vi "Version 1_Write Tare Settings.vi"(6 "Totalizer Timer":enum32{"Disable", "Enable", "No Change"}(radio)=enum."No Change", 8 "error in":errorcluster, 9 "ValveDrive Report":enum32{"Disable", "Enable", "No Change"}(radio)=enum."No Change", 10 "Tare Functions":T1={"Display"=enum."None", "External"=enum."None", "Auto Delay"=nan} {"Auto Delay" format="%.1g"}, 11 "VISA Session In":refnum<visa-resource-name>="Alicat") -> (0 "error out":errorcluster, 3 "VISA Session Out":refnum<visa-resource-name>)   [LabVIEW 2015]
panel:
  in  "Address (A)":string="A"
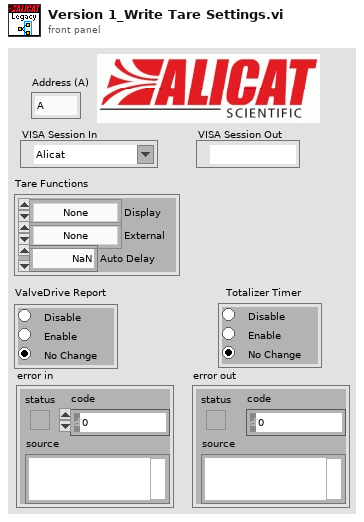
[diagram p1: front panel]
types:
  T1 = cluster{"Display":enum16{"None", "Pressure", "Volumetric"}, "External":enum16{"None", "Pressure", "Volumetric", "Totalizer"}, "Auto Delay":dbl}
  T2 = cluster{"Valve Drive":bool, "Totalizer":bool, "Totalizer Timer":bool, "Totalizer Peak Flow":bool, "Show Abs., Gauge\nand Baro. pressures":bool}
  T3 = cluster{"Pressure(s)":bool, "Temperature":bool, "Volumetric":bool, "Mass":bool, "Totalizer Average Flow":bool, "Gas Selected":bool}
  T4 = cluster{"Absolute Pressure":bool, "Gauge/Diff. Pressure":bool, "Barometric Pressure":bool, "Temperature":bool, "Volumetric":bool, "Mass":bool, "Setpoint":bool, "Valve Drive":bool, "Totalizer":bool, "Totalizer Timer":bool, "Totalizer Average Flow":bool, "Totalizer Peak Flow":bool, "Gas Selected":bool, "Tot. Timer Format":u16}
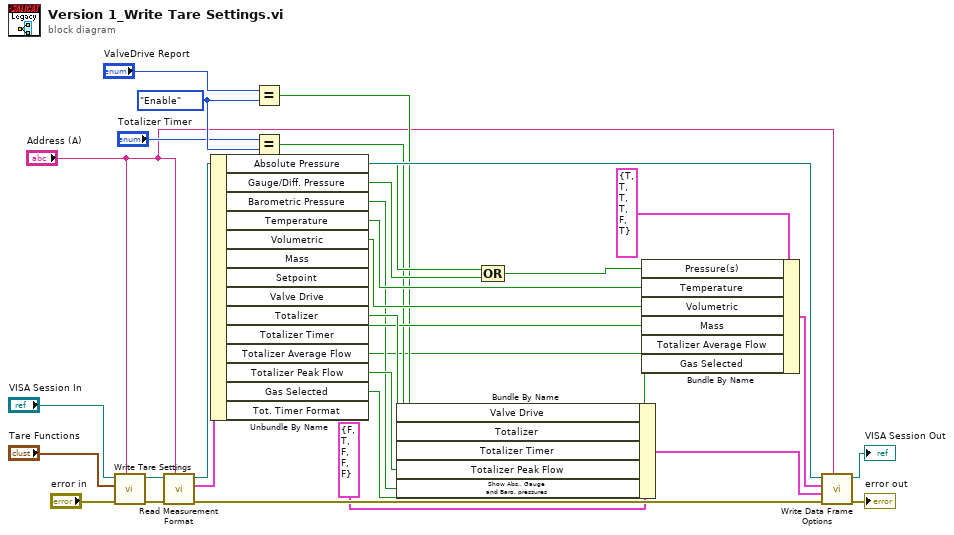
[diagram p0: block diagram]
diagram:
  w9 = enum32{"Disable", "Enable", "No Change"}."Enable" ("Totalizer Timer")
  n1 = call "Write Tare Settings.vi"("Unit ID (A)"="Address (A)", "error in"="error in", "Tare Functions"="Tare Functions", "VISA Session In"="VISA Session In") -> ("error out"=w27:errorcluster, "VISA Session Out"=w28:refnum<visa-resource-name>)  [unwired: 6 in]
  n2 = call "Read Measurement Format.vi"("Unit ID (A)"="Address (A)", "error in"=w27, "VISA Session In"=w28) -> ("error out"=w23:errorcluster, "Data Frame Format"=w22:T4, "VISA Session Out"=w26:refnum<visa-resource-name>)  [unwired: 6 in]
  n3 = Unbundle By Name(w22) -> ("Absolute Pressure"=w12:bool, "Gauge/Diff. Pressure"=w13:bool, "Barometric Pressure"=w10:bool, "Temperature"=w14:bool, "Volumetric"=w15:bool, "Mass"=w16:bool, "Totalizer"=w17:bool, "Totalizer Average Flow"=w1:bool, "Totalizer Peak Flow"=w18:bool, "Gas Selected"=w19:bool)  [unwired: 4 out]
  n4 = Equal?(x="ValveDrive Report", y=w9) -> (x = y?=w6:bool)
  n5 = Equal?(x="Totalizer Timer", y=w9) -> (x = y?=w5:bool)
  n6 = Bundle By Name(cluster=T2 {"Valve Drive"=FALSE, "Totalizer"=TRUE, "Totalizer Timer"=FALSE, "Totalizer Peak Flow"=FALSE, "Show Abs., Gauge\nand Baro. pressures"=FALSE} ("Enables: Data frame only"), "Valve Drive"=w6, "Totalizer"=w17, "Totalizer Timer"=w5, "Totalizer Peak Flow"=w18, "Show Abs., Gauge\nand Baro. pressures"=w10) -> (w4:T2)
  n7 = Compound Arithmetic op=OR(w12, w13) -> (w11:bool)
  n8 = Bundle By Name(cluster=T3 {"Pressure(s)"=TRUE, "Temperature"=TRUE, "Volumetric"=TRUE, "Mass"=TRUE, "Totalizer Average Flow"=FALSE, "Gas Selected"=TRUE} ("Enables: \nData frame and Display"), "Pressure(s)"=w11, "Temperature"=w14, "Volumetric"=w15, "Mass"=w16, "Totalizer Average Flow"=w1, "Gas Selected"=w19) -> (w3:T3)
  n9 = call "Write Data Frame Options.vi"("Unit ID (A)"="Address (A)", "error in"=w23, "Enables: Data frame only"=w4, "Enables: \nData frame and Display"=w3, "VISA Session In"=w26) -> ("error out"=→"error out":errorcluster, "VISA Session Out"=→"VISA Session Out":refnum<visa-resource-name>)  [unwired: 5 in]
